vi "Is Initialized.vi"(8 "error in":errorcluster, 11 "Virtual Thermometer in":refnum<class "Virtual Thermometer.lvclass">) -> (0 "error out":errorcluster, 2 "Is Initialized?":bool, 3 "Virtual Thermometer out":refnum<class "Virtual Thermometer.lvclass">)   [LabVIEW 2024, in "Virtual Thermometer.lvclass"]
uses:
  Virtual Thermometer.lvclass
  Virtual Thermometer.lvclass/Virtual Thermometer.ctl
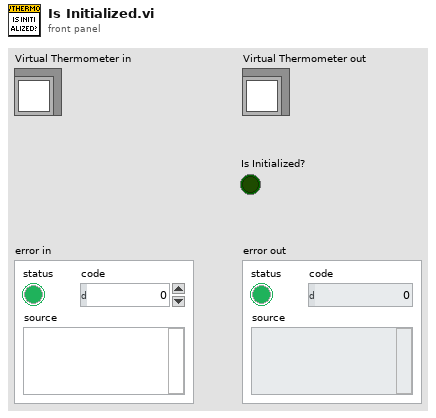
[diagram p1: front panel]
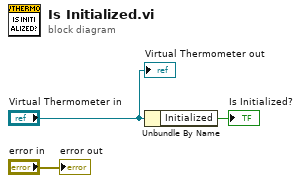
[diagram p0: block diagram]
diagram:
  n1 = Unbundle By Name("Virtual Thermometer in") -> ("Initialized"=→"Is Initialized?":bool)
  "Virtual Thermometer out" <- "Virtual Thermometer in"
  "error out" <- "error in"
